vi "dfd_CIC_CombStage.vi"(10 "input valid":bool, 11 "data in":bool[](array[boolean])) -> (2 "output valid":bool, 3 "data out":bool[](array[boolean]))   [LabVIEW 2017]
uses:
  <vilib>/rvi/FXPMathLib/basic elements/FxpDiscreteDelay/XNode/nifxpmath_DiscreteDelay.xnode
  <vilib>/rvi/FXPMathLib/basic elements/FxpAddSub/XNode/nifxpmath_AddSub.xnode
  <vilib>/rvi/FXPMathLib/sim/FxpSim.dll
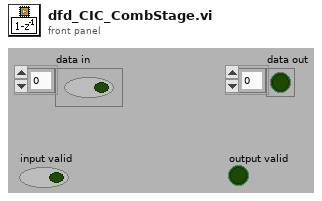
[diagram p1: front panel]
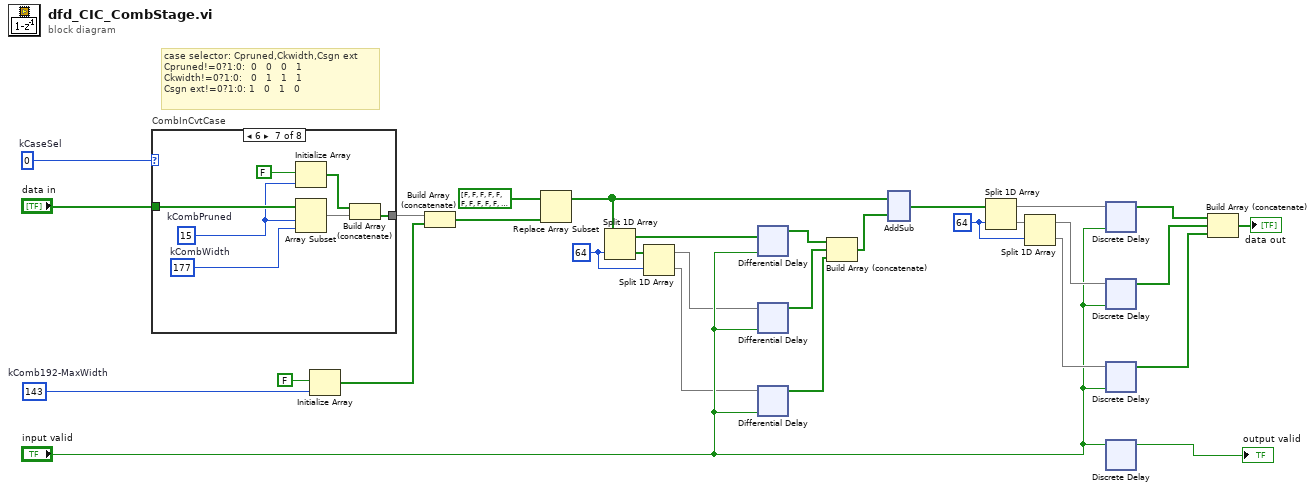
[diagram p0: block diagram]
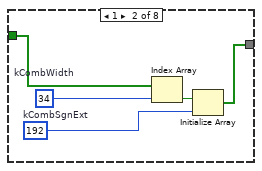
[diagram p3: hidden frame]
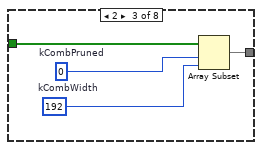
[diagram p4: hidden frame]
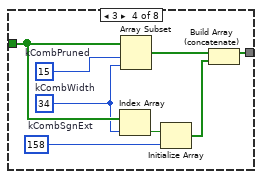
[diagram p5: hidden frame]
diagram:
  w21 = 64 ("index")
  w23 = 143  # kComb192-MaxWidth
  w5 = 0  # kCaseSel
  w29 = 64 ("index")
  # "case selector: Cpruned,Ckwidth,Csgn ext\nCpruned!=0?1:0:  0   0   0   1\nCkwidth!=0?1:0:   0   1   1   1\nCsgn ext!=0?1:0: 1   0   1   0"
  n1 = case "CombInCvtCase" shown="6" w5 {
    tunnel: "data in" -> [w31 w36 w40 w48 w49 w50 w57 w58]
    tunnel: [w31 w34 w39 w44 w49 w50 w53 w58] -> w7
    frame 0, Default {
    }
    frame 1 {
      w32 = 192  # kCombSgnExt
      w33 = 34  # kCombWidth
      n2 = Index Array(array=w36, index=w33) -> (element=w35:bool)
      n3 = Initialize Array(w35, w32) -> (w34:bool[])
    }
    frame 2 {
      w37 = 192  # kCombWidth
      w38 = 0  # kCombPruned
      n4 = Array Subset(array=w40, index=w38, length=w37) -> (w39:bool[])
    }
    frame 3 {
      w41 = 158  # kCombSgnExt
      w42 = 34  # kCombWidth
      w43 = 15  # kCombPruned
      n5 = Index Array(array=w48, index=w42) -> (element=w45:bool)
      n6 = Array Subset(array=w48, index=w43, length=w42) -> (w47:bool[])
      n7 = Initialize Array(w45, w41) -> (w46:bool[])
      n8 = Build Array (concatenate)(w47, w46) -> (w44:bool[])
    }
    frame 4 {
    }
    frame 5 {
    }
    frame 6 {
      w51 = 177  # kCombWidth
      w52 = 15  # kCombPruned
      n9 = Initialize Array(FALSE, w52) -> (w54:bool[])
      n10 = Array Subset(array=w57, index=w52, length=w51) -> (w56:bool[])
      n11 = Build Array (concatenate)(w54, w56) -> (w53:bool[])
    }
    frame 7 {
    }
  }
  n12 = Initialize Array(FALSE, w23) -> (w6:bool[])
  n13 = Build Array (concatenate)(w7, w6) -> (w2:bool[])
  n14 = Replace Array Subset(array=bool[] [FALSE, FALSE, FALSE, FALSE, FALSE, FALSE, FALSE, FALSE, FALSE, FALSE, FALSE, FALSE, FALSE, FALSE, FALSE, FALSE, FALSE, FALSE, FALSE, FALSE, FALSE, FALSE, FALSE, FALSE, FALSE, FALSE, FALSE, FALSE, FALSE, FALSE, FALSE, FALSE, FALSE, FALSE, FALSE, FALSE, FALSE, FALSE, FALSE, FALSE, FALSE, FALSE, FALSE, FALSE, FALSE, FALSE, FALSE, FALSE, FALSE, FALSE, FALSE, FALSE, FALSE, FALSE, FALSE, FALSE, FALSE, FALSE, FALSE, FALSE, FALSE, FALSE, FALSE, FALSE, FALSE, FALSE, FALSE, FALSE, FALSE, FALSE, FALSE, FALSE, FALSE, FALSE, FALSE, FALSE, FALSE, FALSE, FALSE, FALSE, FALSE, FALSE, FALSE, FALSE, FALSE, FALSE, FALSE, FALSE, FALSE, FALSE, FALSE, FALSE, FALSE, FALSE, FALSE, FALSE, FALSE, FALSE, FALSE, FALSE, FALSE, FALSE, FALSE, FALSE, FALSE, FALSE, FALSE, FALSE, FALSE, FALSE, FALSE, FALSE, FALSE, FALSE, FALSE, FALSE, FALSE, FALSE, FALSE, FALSE, FALSE, FALSE, FALSE, FALSE, FALSE, FALSE, FALSE, FALSE, FALSE, FALSE, FALSE, FALSE, FALSE, FALSE, FALSE, FALSE, FALSE, FALSE, FALSE, FALSE, FALSE, FALSE, FALSE, FALSE, FALSE, FALSE, FALSE, FALSE, FALSE, FALSE, FALSE, FALSE, FALSE, FALSE, FALSE, FALSE, FALSE, FALSE, FALSE, FALSE, FALSE, FALSE, FALSE, FALSE, FALSE, FALSE, FALSE, FALSE, FALSE, FALSE, FALSE, FALSE, FALSE, FALSE, FALSE, FALSE, FALSE, FALSE, FALSE, FALSE, FALSE, FALSE, FALSE, FALSE, FALSE, FALSE, FALSE, FALSE, FALSE, FALSE, TRUE, TRUE] ("Array"), new element=w2) -> (w1:bool[])  [unwired: 1 in]
  n15 = Split 1D Array(array=w1, index=w29) -> (first subarray=w10:bool[], second subarray=w28:bool[])
  n16 = Split 1D Array(array=w28, index=w29) -> (first subarray=w9:bool[], second subarray=w4:bool[])
  n17 = xnode ("Differential Delay")("D"=w10, "enable"="input valid") -> ("Q"=w26:bool[])
  n18 = xnode ("Differential Delay")("D"=w9, "enable"="input valid") -> ("Q"=w27:bool[])
  n19 = xnode ("Differential Delay")("D"=w4, "enable"="input valid") -> ("Q"=w30:bool[])
  n20 = Build Array (concatenate)(w26, w27, w30) -> (w25:bool[])
  n21 = xnode ("AddSub")("x"=w1, "y"=w25) -> ("s"=w14:bool[])  [unwired: 1 out]
  n22 = Split 1D Array(array=w14, index=w21) -> (first subarray=w17:bool[], second subarray=w20:bool[])
  n23 = Split 1D Array(array=w20, index=w21) -> (first subarray=w16:bool[], second subarray=w15:bool[])
  n24 = xnode ("Discrete Delay")("D"=w17, "enable"="input valid") -> ("Q"=w18:bool[])
  n25 = xnode ("Discrete Delay")("D"=w16, "enable"="input valid") -> ("Q"=w19:bool[])
  n26 = xnode ("Discrete Delay")("D"=w15, "enable"="input valid") -> ("Q"=w22:bool[])
  n27 = xnode ("Discrete Delay")("D"="input valid") -> ("Q"=→"output valid":bool)
  n28 = Build Array (concatenate)(w18, w19, w22) -> (→"data out":bool[])
